vi "JKISM++ Switch VI Description Language Tool.vi"() -> ()   [LabVIEW 2014]
panel:
  in  "Double Click To Run...":i32(listbox)=-1
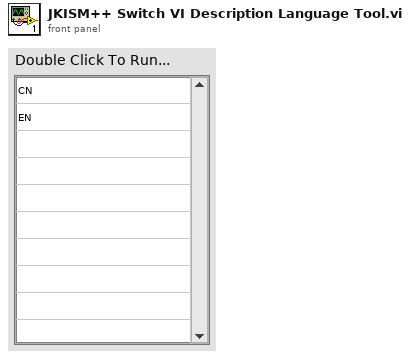
[diagram p1: front panel]
types:
  T1 = enum32{"Invalid", "Standard", "Closed", "Hidden", "Minimized", "Maximized"}
  T2 = enum32{"invalid app kind", "Development System", "Run Time System", "Student Edition", "Embedded LabVIEW", "Evaluation", "Custom"}
  T3 = cluster{"Core":cluster{"Current VI Reference":refnum<vi>, "Close Panel on Exit?":bool}, "Your Boolean data":bool, "Language":string[], "Help Root":path}
  T4 = cluster{"Current VI Reference":refnum<vi>, "Close Panel on Exit?":bool}
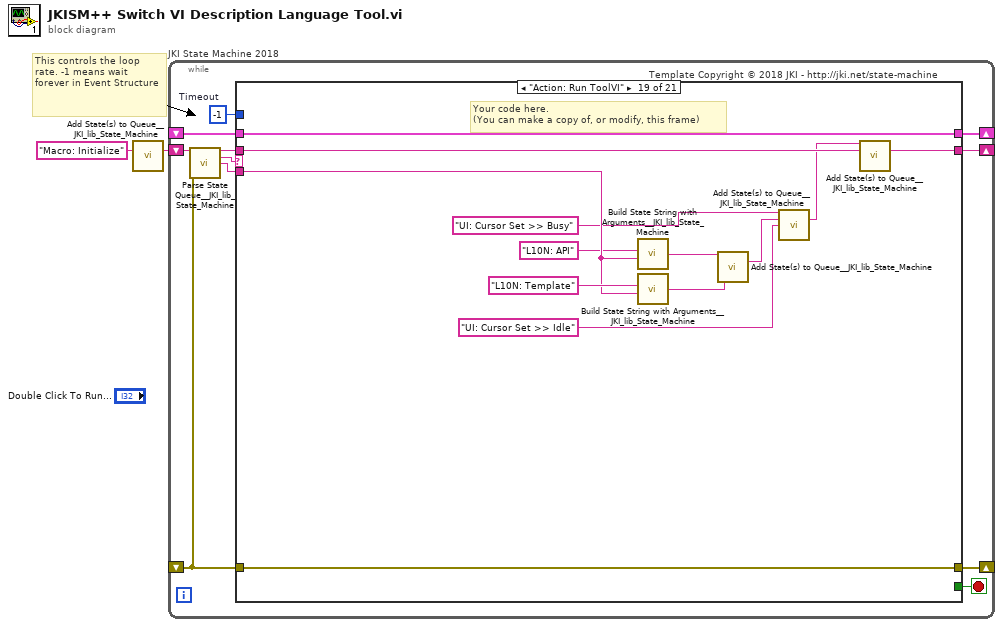
[diagram p0: block diagram]
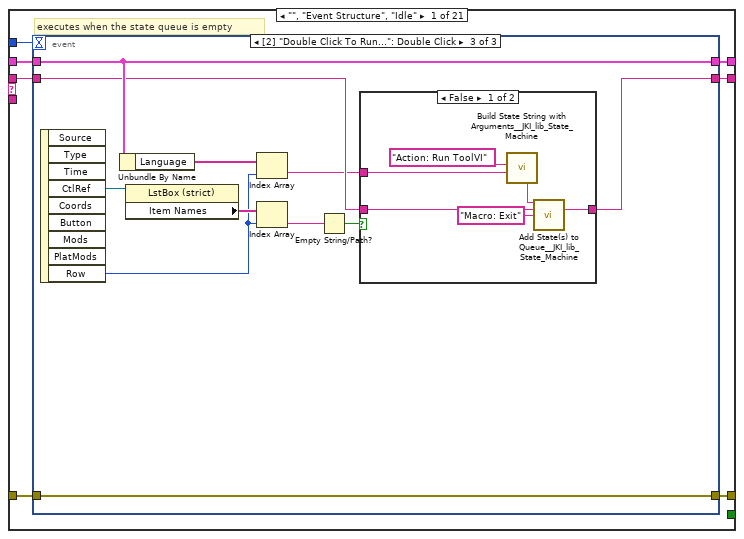
[diagram p2: hidden frame]
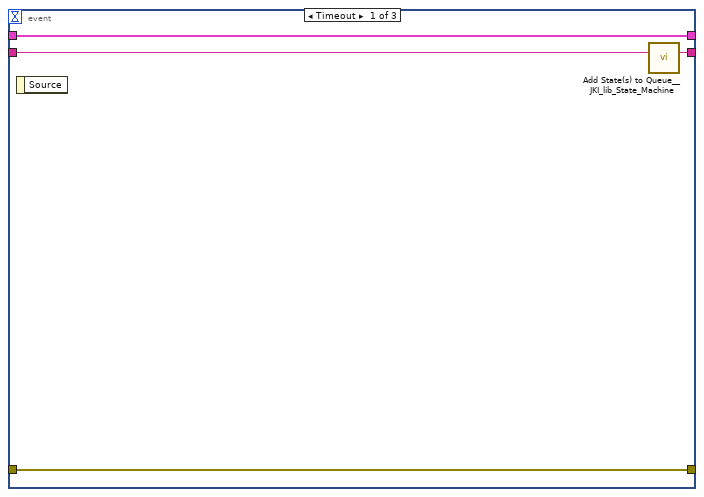
[diagram p3: hidden frame]
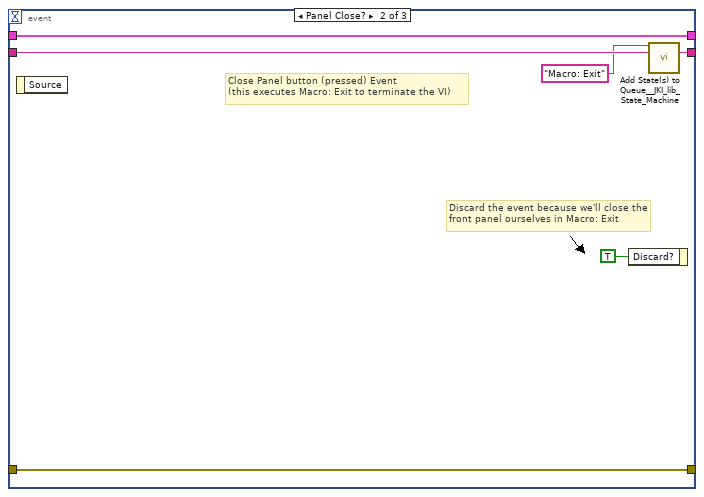
[diagram p4: hidden frame]
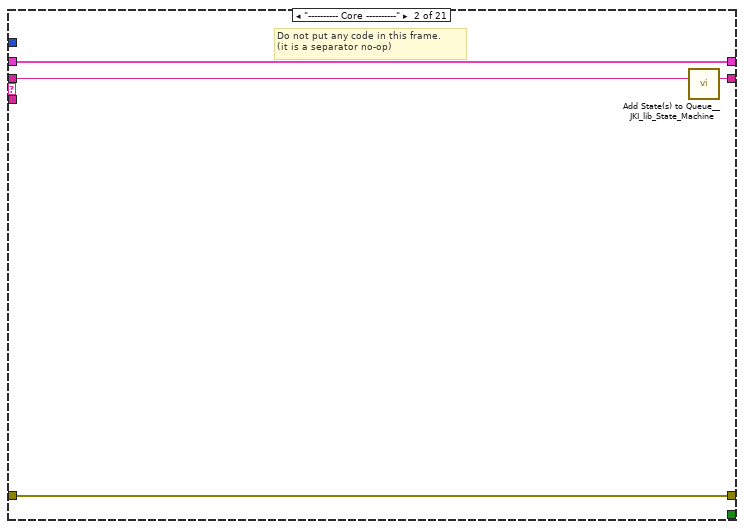
[diagram p6: hidden frame]
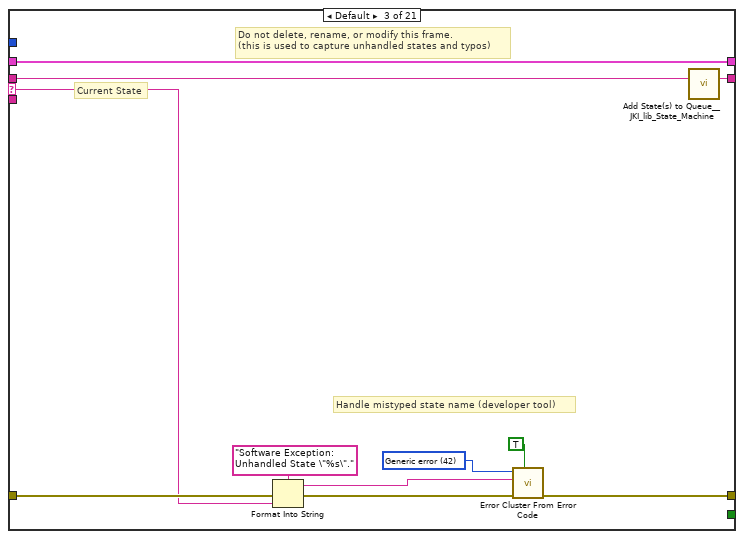
[diagram p7: hidden frame]
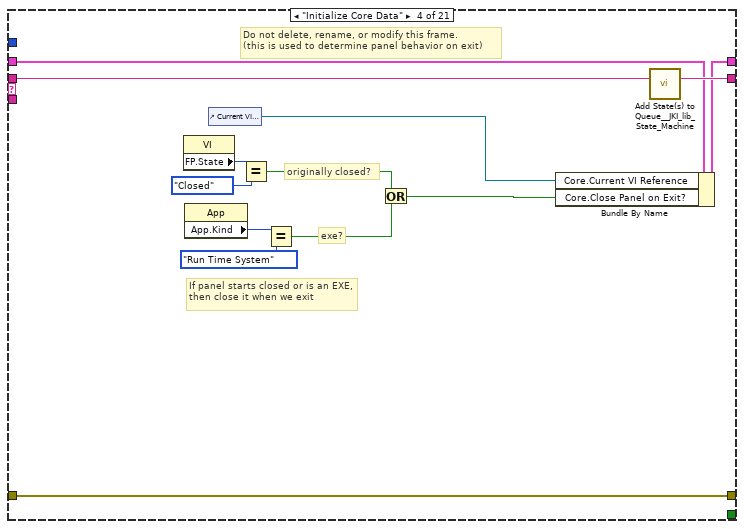
[diagram p8: hidden frame]
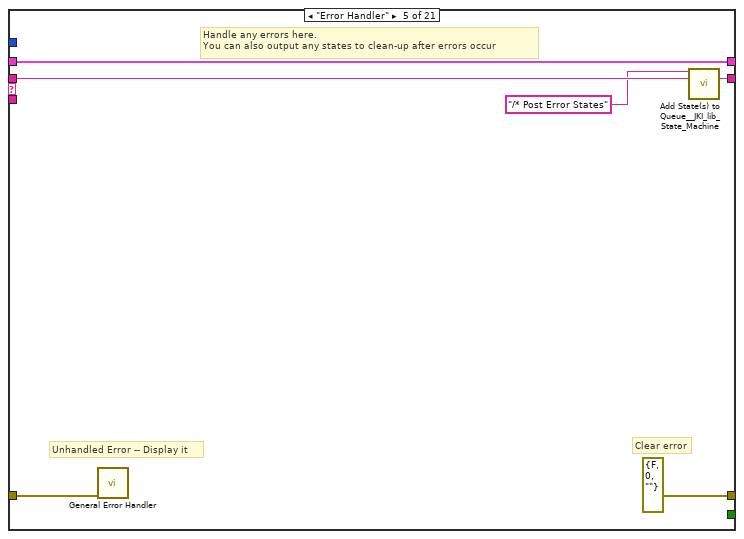
[diagram p9: hidden frame]
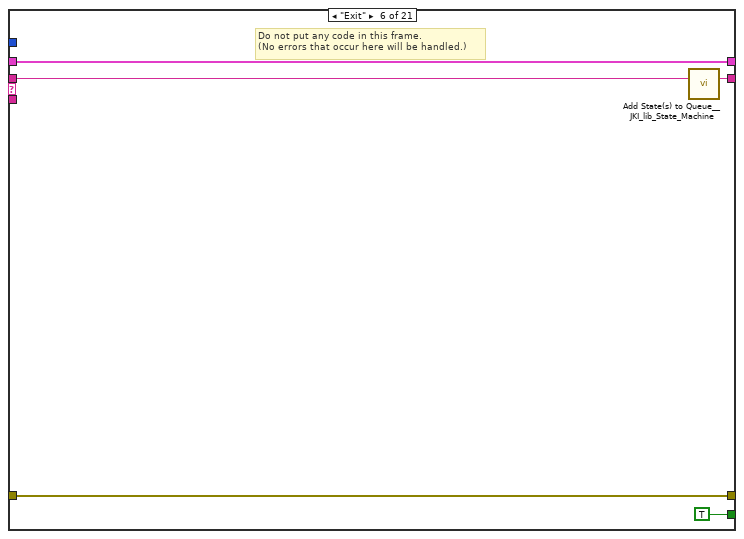
[diagram p10: hidden frame]
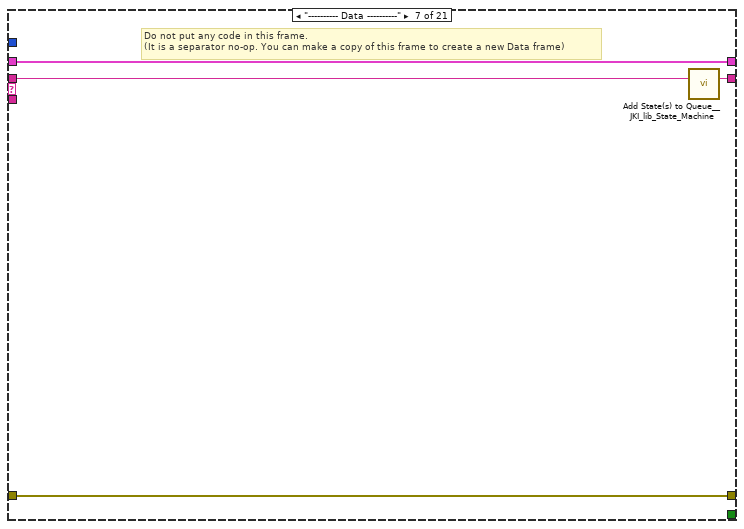
[diagram p11: hidden frame]
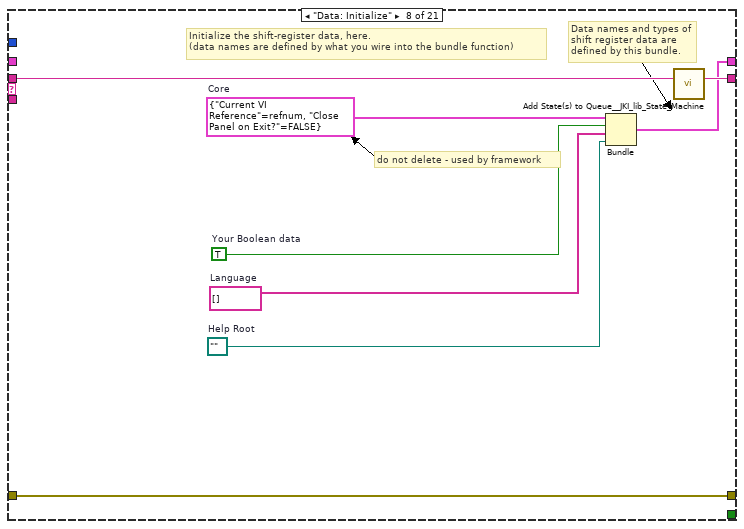
[diagram p12: hidden frame]
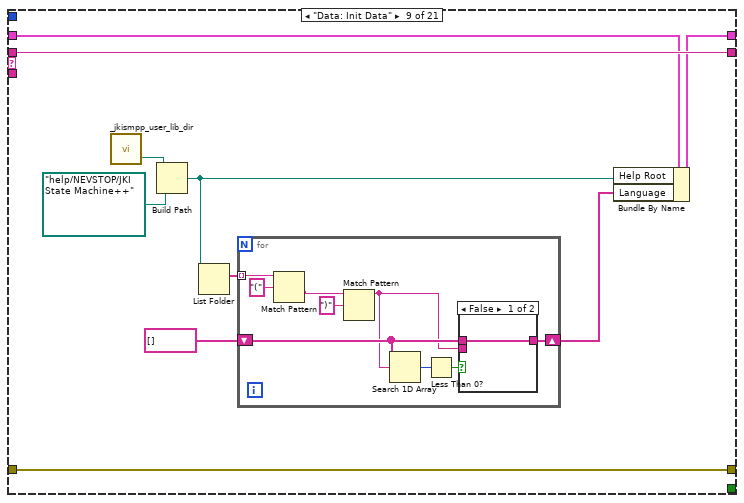
[diagram p13: hidden frame]
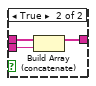
[diagram p14: hidden frame]
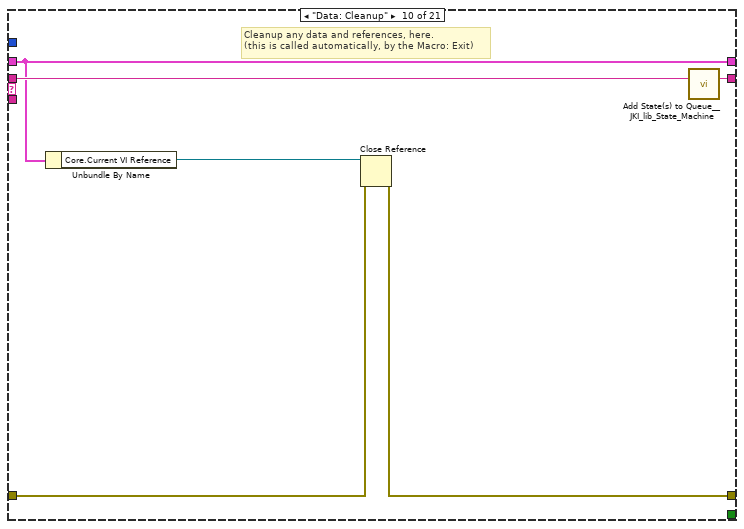
[diagram p15: hidden frame]
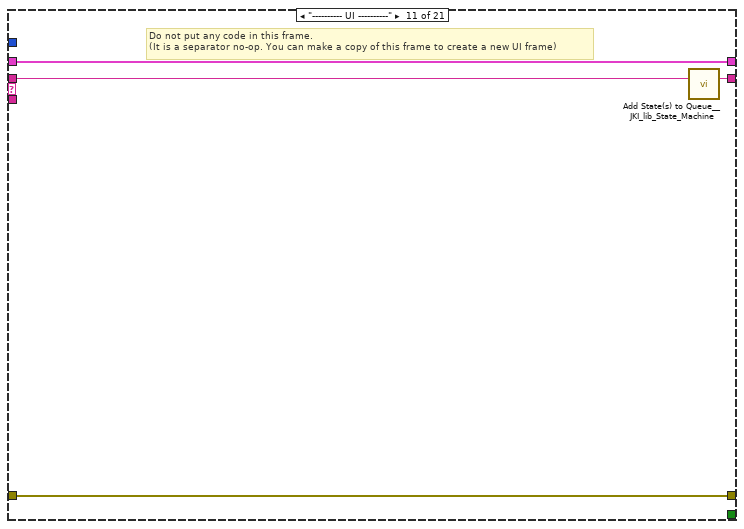
[diagram p16: hidden frame]
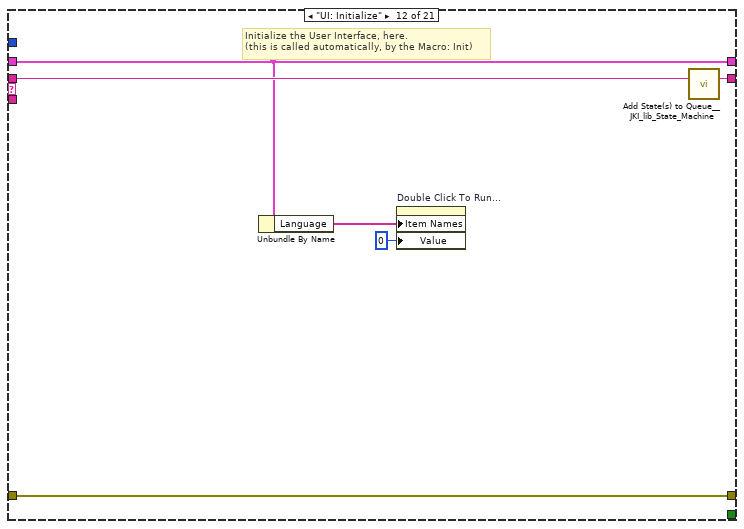
[diagram p17: hidden frame]
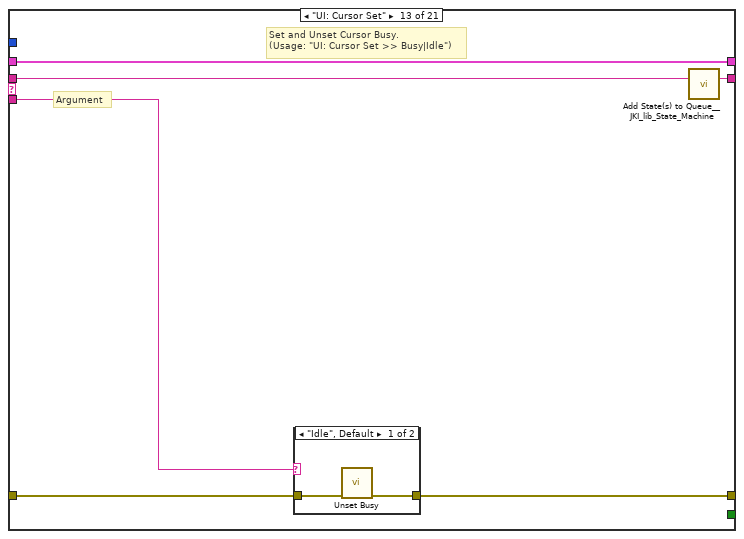
[diagram p18: hidden frame]
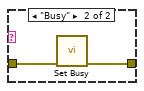
[diagram p19: hidden frame]
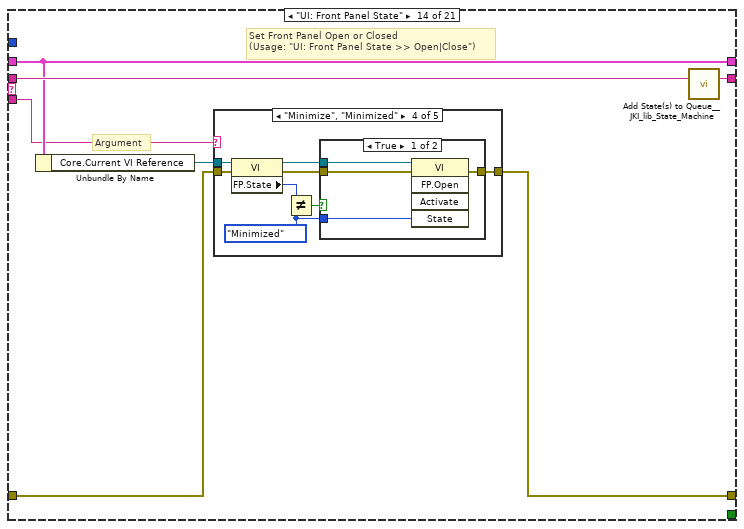
[diagram p20: hidden frame]
diagram:
  # "This controls the loop rate. -1 means wait forever in Event Structure"
  n1 = call <vilib>:"Add State(s) to Queue__JKI_lib_State_Machine.vi"("State(s) in (\"\")"="Macro: Initialize") -> ("States Out"=w2:string)  [unwired: 14 in]
  n2 = while "JKI State Machine 2018" {
    shift-right: [w6] -> _
    shift-left: _ -> [w5]
    shift-right: [w9] -> _
    shift-left: _ -> [w3]
    shift-right: [w8] -> _
    shift-left: w2 -> [w10]
    stop <- w7 stop-if-true
    w4 = -1  # Timeout
    # "Template Copyright © 2018 JKI - http://jki.net/state-machine"
    n3 = call <vilib>:"Parse State Queue__JKI_lib_State_Machine.vi"("State Queue"=w10, "Error In (no error)"=w3) -> ("Remaining States"=w12:string, "Current State"=w13:string, "Arguments"=w11:string)  [unwired: 11 in]
    n4 = case shown="\"Action: Run ToolVI\"" w13 {
      selector: w13 -> [_ _ w53 _ _ _ _ _ _ _ _ _ _ _ _ _ _ _ _ _ _]
      tunnel: w12 -> [w20 w52 w57 w76 w82 w87 w91 w99 w108 w128 w132 w138 w144 w155 w224 w229 w239 w243 w256 w266 w277]
      tunnel: w11 -> [_ _ _ _ _ _ _ _ _ _ _ _ w139 w149 _ _ _ _ w249 w257 w268]
      tunnel: w5 -> [w18 w49 w55 w69 w79 w85 w88 _ w107 w123 w129 w135 w142 w151 w221 w226 w236 w240 w254 w260 w276]
      tunnel: [w17 w50 w59 w73 errorcluster {"status"=FALSE, "code"=0, "source"=""} ("error out") w84 w89 w96 w109 w124 w130 w136 w140 w152 w222 w227 w237 w241 w253 w267 w278] -> w9
      tunnel: w3 -> [w16 w50 w58 w73 w78 w84 w89 w96 w109 w125 w130 w136 w141 w153 w222 w227 w237 w241 w253 w267 w278]
      tunnel: [w19 w51 w56 w75 w81 w86 w90 w98 w108 w127 w131 w137 w143 w154 w223 w228 w238 w242 w255 w266 w277] -> w8
      tunnel: [_ _ _ _ _ TRUE _ _ _ _ _ _ _ _ _ _ _ _ _ _ _] -> w7
      tunnel: [w15 w49 w55 w74 w79 w85 w88 w97 w106 w123 w129 w135 w142 w151 w221 w226 w236 w240 w254 w260 w276] -> w6
      tunnel: w4 -> [w14 _ _ _ _ _ _ _ _ _ _ _ _ _ _ _ _ _ _ _ _]
      frame "", "Event Structure", "Idle" {
        # "executes when the state queue is empty"
        n5 = event shown="[2] \"Double Click To Run...\": Double Click" {
          selector: _ -> [_ _ _]
          dyn-events: _ -> [_ _ _]
          timeout: w14 -> [_ _ _]
          tunnel: w20 -> [w24 w30 w35]
          tunnel: [w23 w29 w34] -> w19
          tunnel: w18 -> [w21 w27 w38]
          tunnel: [w22 w28 w41] -> w17
          tunnel: w16 -> [w22 w28 w41]
          tunnel: [w21 w27 w38] -> w15
          event Timeout {
            n6 = event-data() -> ()  [unwired: 1 in, 1 out]
            n7 = call <vilib>:"Add State(s) to Queue__JKI_lib_State_Machine.vi"("State(s) in (\"\")"=w24) -> ("States Out"=w23:string)  [unwired: 14 in]
          }
          event Panel Close? {
            # "Discard the event because we'll close the front panel ourselves in Macro: Exit"
            # "Close Panel button (pressed) Event\n(this executes Macro: Exit to terminate the VI)"
            n8 = event-data() -> ()  [unwired: 1 in, 1 out]
            n9 = event-data("Discard?"=TRUE) -> ()  [unwired: 1 in, 1 out]
            n10 = call <vilib>:"Add State(s) to Queue__JKI_lib_State_Machine.vi"("State(s) in Front (\"\")"="Macro: Exit", "State(s) in (\"\")"=w30) -> ("States Out"=w29:string)  [unwired: 13 in]
          }
          event "Double Click To Run...": Double Click {
            n11 = event-data() -> ("CtlRef"=w40:refnum<vi>, "Row"=w36:i32)  [unwired: 1 in, 7 out]
            n12 = Unbundle By Name(w38) -> ("Language"=w37:string[])
            n13 = property class="LstBox (strict)"(reference=w40) -> ("Item Names"=w39:string[])  [unwired: 1 in, 2 out]
            n14 = Index Array(array=w37, index=w36) -> (element=w31:string)
            n15 = Index Array(array=w39, index=w36) -> (element=w33:string)
            n16 = Empty String/Path?(string/path=w33) -> (empty?=w32:bool)
            n17 = case shown="False" w32 {
              tunnel: w35 -> [w47 w48]
              tunnel: [w46 w48] -> w34
              tunnel: w31 -> [w42 _]
              frame False {
                n18 = call <vilib>:"Build State String with Arguments__JKI_lib_State_Machine.vi"("Arguments (\"\")"=w42, "State"="Action: Run ToolVI") -> ("State with Arguments"=w44:string)  [unwired: 4 in]
                n19 = call <vilib>:"Add State(s) to Queue__JKI_lib_State_Machine.vi"("State(s) in Front (\"\")"=w44, "State(s) in (\"\")"=w47, "State(s) at Back (\"\")"="Macro: Exit" ("State(s) at Back (\"\")")) -> ("States Out"=w46:string)  [unwired: 12 in]
              }
              frame True {
              }
            }
          }
        }
      }
      frame "---------- Core ----------" {
        # "Do not put any code in this frame.\n(it is a separator no-op)"
        n20 = call <vilib>:"Add State(s) to Queue__JKI_lib_State_Machine.vi"("State(s) in (\"\")"=w52) -> ("States Out"=w51:string)  [unwired: 14 in]
      }
      frame Default {
        w62 = 42 items=["No error", "Argument error", "Memory is full", "Out of zone", "End of file", "File already open", "Generic file I/O error", "File not found", "File permission error", "Disk is full", "Duplicate path", "Too many files open", "System feature not enabled", "Resource file not found", "Cannot add resource", "Resource not found", "Image not found", "Image memory error", "Pen does not exist", "Config type invalid", "Config token not found", "Config parse error", "Config memory error", "Bad external code format", "Bad external code offset", "External code not present", "Null window", "Destroy window error", "Null menu", "Print aborted", "Bad print record", "Print driver error", "Windows error during printing", "Memory error during printing", "Print dialog error", "Generic print error", "Invalid device refnum", "Device not found", "Device parameter error", "Device unit error", "Cannot open device", "Device call aborted", "Generic error", "Cancelled by user", "Object ID too low", "Object ID too high", "Object not in heap", "Unknown heap", "Unknown object (invalid DefProc)", "Unknown object (DefProc not in table)", "Message out of range", "Invalid (null) method", "Unknown message", "Manager call not supported", "Bad address", "Network operation in progress", "Network operation timed out", "Connection is busy", "Network attribute not supported", "Network error", "Address in use", "System out of memory", "Connection aborted", "Connection refused", "Not connected", "Already connected", "Connection closed", "Initialization error (interapplication manager)", "Bad occurrence", "Wait on unbound occurrence handler", "Occurrence queue overflow", "Datalog type conflict", "Unused", "Unrecognized type (interapplication manager)", "Memory corrupt", "Failed to make temporary DLL", "Old CIN version", "Drag socket not found", "Failed to load drop-object", "Failed to register OLE object", "Failed to release OLE object", "Format specifier type mismatch", "Unknown format specifier", "Too few format specifiers", "Too many format specifiers", "Scan failed", "Newer CIN version", "Error converting to variant", "Runtime menu error", "Password tampered", "Variant attribute not found", "Incompatible variant data type", "Event data is not available", "Event Store is not present", "Occurrence is not found", "Event Queue is not created", "Event info is not available", "Refnum passed is NULL", "Error retrieving Class GUID", "Error retrieving CoClass GUID", "Error retrieving TypeLib GUID.", "Bad built application magic bytes.", "Specific driver is different from the specific driver associated with the Logical Name.", "There is no session opened to the class driver.", "Max Error", "MAX - Error with config objects", "MAX - Error loading configuration", "MAX - Group not supported"]
        # "Current State"
        # "Do not delete, rename, or modify this frame.\n(this is used to capture unhandled states and typos)"
        # "Handle mistyped state name (developer tool)"
        n21 = Format Into String(format string="Software Exception: Unhandled State \"%s\"." ("message"), error in=w58, w53) -> (resulting string=w61:string, error out=w60:errorcluster)  [unwired: 1 in]
        n22 = call <vilib>:"Error Cluster From Error Code.vi"("show call chain? (False)"=TRUE, "error in (no error)"=w60, "error message (\"\")"=w61, "error code (0)"=w62) -> ("error out"=w59:errorcluster)  [unwired: 5 in]
        n23 = call <vilib>:"Add State(s) to Queue__JKI_lib_State_Machine.vi"("State(s) in (\"\")"=w57) -> ("States Out"=w56:string)  [unwired: 14 in]
      }
      frame "Initialize Core Data" {
        # "Do not delete, rename, or modify this frame.\n(this is used to determine panel behavior on exit)"
        # "originally closed?"
        # "exe?"
        # "If panel starts closed or is an EXE, then close it when we exit"
        n24 = property class="VI"() -> ("FP.State"=w66:T1)  [unwired: 2 in, 2 out]
        n25 = property class="App"() -> ("App.Kind"=w72:T2)  [unwired: 2 in, 2 out]
        n26 = control-ref of="Current VI Reference"() -> (w67:refnum<vi>)
        n27 = Equal?(x=w66, y=T1."Closed" ("Front Panel Window:State")) -> (x = y?=w64:bool)
        n28 = Equal?(x=w72, y=T2."Run Time System" ("Application:Kind")) -> (x = y?=w70:bool)
        n29 = Or(x=w64, y=w70) -> (x .or. y?=w68:bool)
        n30 = Bundle By Name(cluster=w69, "Core.Current VI Reference"=w67, "Core.Close Panel on Exit?"=w68) -> (w74:T3)
        n31 = call <vilib>:"Add State(s) to Queue__JKI_lib_State_Machine.vi"("State(s) in (\"\")"=w76) -> ("States Out"=w75:string)  [unwired: 14 in]
      }
      frame "Error Handler" {
        # "Unhandled Error -- Display it"
        # "Handle any errors here.\nYou can also output any states to clean-up after errors occur"
        # "Clear error"
        n32 = call <vilib>:"General Error Handler.vi"("error in (no error)"=w78) -> ()  [unwired: 10 in, 5 out]
        n33 = call <vilib>:"Add State(s) to Queue__JKI_lib_State_Machine.vi"("State(s) in Front (\"\")"="/* Post Error States", "State(s) in (\"\")"=w82) -> ("States Out"=w81:string)  [unwired: 13 in]
      }
      frame "Exit" {
        # "Do not put any code in this frame.\n(No errors that occur here will be handled.)"
        n34 = call <vilib>:"Add State(s) to Queue__JKI_lib_State_Machine.vi"("State(s) in (\"\")"=w87) -> ("States Out"=w86:string)  [unwired: 14 in]
      }
      frame "---------- Data ----------" {
        # "Do not put any code in this frame.\n(It is a separator no-op. You can make a copy of this frame to create a new Data frame)"
        n35 = call <vilib>:"Add State(s) to Queue__JKI_lib_State_Machine.vi"("State(s) in (\"\")"=w91) -> ("States Out"=w90:string)  [unwired: 14 in]
      }
      frame "Data: Initialize" {
        w92 = string[] []  # Language
        w93 = path ""  # Help Root
        w94 = T4 {"Current VI Reference"=refnum, "Close Panel on Exit?"=FALSE}  # Core
        w95 = TRUE  # Your Boolean data
        # "do not delete - used by framework"
        # "Data names and types of shift register data are defined by this bundle."
        # "Initialize the shift-register data, here.\n(data names are defined by what you wire into the bundle function)"
        n36 = Bundle("Core"=w94, "Your Boolean data"=w95, "Language"=w92, "Help Root"=w93) -> (w97:T3)  [unwired: 1 in]
        n37 = call <vilib>:"Add State(s) to Queue__JKI_lib_State_Machine.vi"("State(s) in (\"\")"=w99) -> ("States Out"=w98:string)  [unwired: 14 in]
      }
      frame "Data: Init Data" {
        n38 = call "_jkismpp_user_lib_dir.vi"() -> ("<LabVIEW>"=w104:path)  [unwired: 2 in, 1 out]
        n39 = Build Path(base path=w104, name or relative path=path "help/NEVSTOP/JKI State Machine++" ("Path")) -> (appended path=w103:path)
        n40 = List Folder(path=w103) -> (filenames=w102:string[])  [unwired: 3 in, 3 out]
        n41 = for {
          tunnel: w102 -> [w118] mode=indexing
          shift-right: [w113] -> w100
          shift-left: string[] [] -> [w114]
          n42 = Match Pattern(string=w118, regular expression="(") -> (after substring=w115:string)  [unwired: 1 in, 3 out]
          n43 = Match Pattern(string=w115, regular expression=")") -> (before substring=w112:string)  [unwired: 1 in, 3 out]
          n44 = Search 1D Array(1D array=w114, element=w112) -> (index of element=w111:i32)  [unwired: 1 in]
          n45 = Less Than 0?(x=w111) -> (x < 0?=w110:bool)
          n46 = case shown="False" w110 {
            tunnel: w114 -> [w119 w122]
            tunnel: [w119 w121] -> w113
            tunnel: w112 -> [_ w120]
            frame False {
            }
            frame True {
              n47 = Build Array (concatenate)(w122, w120) -> (w121:string[])
            }
          }
        }
        n48 = Bundle By Name(cluster=w107, "Help Root"=w103, "Language"=w100) -> (w106:T3)
      }
      frame "Data: Cleanup" {
        # "Cleanup any data and references, here.\n(this is called automatically, by the Macro: Exit)"
        n49 = Unbundle By Name(w123) -> ("Core.Current VI Reference"=w126:refnum<vi>)
        n50 = Close Reference(reference=w126, error in (no error)=w125) -> (error out=w124:errorcluster)
        n51 = call <vilib>:"Add State(s) to Queue__JKI_lib_State_Machine.vi"("State(s) in (\"\")"=w128) -> ("States Out"=w127:string)  [unwired: 14 in]
      }
      frame "---------- UI ----------" {
        # "Do not put any code in this frame.\n(It is a separator no-op. You can make a copy of this frame to create a new UI frame)"
        n52 = call <vilib>:"Add State(s) to Queue__JKI_lib_State_Machine.vi"("State(s) in (\"\")"=w132) -> ("States Out"=w131:string)  [unwired: 14 in]
      }
      frame "UI: Initialize" {
        # "Initialize the User Interface, here.\n(this is called automatically, by the Macro: Init)"
        n53 = Unbundle By Name(w135) -> ("Language"=w134:string[])
        n54 = property on="Double Click To Run..." class="LstBox (strict)"("Item Names"=w134, "Value"=0 ("Double Click To Run...")) -> ()  [unwired: 2 in, 2 out]
        n55 = call <vilib>:"Add State(s) to Queue__JKI_lib_State_Machine.vi"("State(s) in (\"\")"=w138) -> ("States Out"=w137:string)  [unwired: 14 in]
      }
      frame "UI: Cursor Set" {
        # "Argument"
        # "Set and Unset Cursor Busy.\n(Usage: \"UI: Cursor Set >> Busy|Idle\")"
        n56 = case shown="\"Idle\", Default" w139 {
          tunnel: w141 -> [w146 w148]
          tunnel: [w145 w147] -> w140
          frame "Idle", Default {
            n57 = call <vilib>:"Unset Busy.vi"("error in (no error)"=w146) -> ("error out"=w145:errorcluster)  [unwired: 10 in]
          }
          frame "Busy" {
            n58 = call <vilib>:"Set Busy.vi"("error in (no error)"=w148) -> ("error out"=w147:errorcluster)  [unwired: 9 in, 1 out]
          }
        }
        n59 = call <vilib>:"Add State(s) to Queue__JKI_lib_State_Machine.vi"("State(s) in (\"\")"=w144) -> ("States Out"=w143:string)  [unwired: 14 in]
      }
      frame "UI: Front Panel State" {
        # "Argument"
        # "Set Front Panel Open or Closed\n(Usage: \"UI: Front Panel State >> Open|Close\")"
        n60 = Unbundle By Name(w151) -> ("Core.Current VI Reference"=w150:refnum<vi>)
        n61 = case shown="\"Minimize\", \"Minimized\"" w149 {
          tunnel: w153 -> [w161 w176 w187 w200 w213]
          tunnel: [w163 w177 w189 w202 w215] -> w152
          tunnel: w150 -> [w162 w174 w188 w201 w214]
          frame "Open", "Standard", Default {
            w156 = T1."Standard" ("State")
            n62 = property class="VI"(reference=w162, error in=w161) -> (reference out=w159:refnum<vi>, error out=w160:errorcluster, "FP.State"=w158:T1)
            n63 = Not Equal?(x=w158, y=w156) -> (x != y?=w157:bool)
            n64 = case shown="True" w157 {
              tunnel: [w167 w169] -> w163
              tunnel: w160 -> [w166 w169]
              tunnel: w159 -> [w165 _]
              tunnel: w156 -> [w164 _]
              frame True {
                n65 = invoke class="VI" method="FP.Open"(reference=w165, error in=w166, "Activate"=TRUE, "State"=w164) -> (error out=w167:errorcluster)  [unwired: 1 in, 4 out]
              }
              frame False {
              }
            }
          }
          frame "Close", "Closed" {
            n66 = property class="VI"(reference=w174, error in=w176) -> (reference out=w173:refnum<vi>, error out=w175:errorcluster, "FP.State"=w171:T1)
            n67 = Not Equal?(x=w171, y=T1."Closed" ("Front Panel Window:State")) -> (x != y?=w170:bool)
            n68 = case shown="True" w170 {
              tunnel: [w178 w181] -> w177
              tunnel: w175 -> [w178 w180]
              tunnel: w173 -> [_ w179]
              frame False {
              }
              frame True {
                n69 = invoke class="VI" method="FP.Close"(reference=w179, error in=w180) -> (error out=w181:errorcluster)  [unwired: 1 in, 2 out]
              }
            }
          }
          frame "Hidden", "Hide" {
            w182 = T1."Hidden" ("State")
            n70 = property class="VI"(reference=w188, error in=w187) -> (reference out=w185:refnum<vi>, error out=w186:errorcluster, "FP.State"=w184:T1)
            n71 = Not Equal?(x=w184, y=w182) -> (x != y?=w183:bool)
            n72 = case shown="True" w183 {
              tunnel: [w193 w194] -> w189
              tunnel: w186 -> [w192 w194]
              tunnel: w185 -> [w191 _]
              tunnel: w182 -> [w190 _]
              frame True {
                n73 = invoke class="VI" method="FP.Open"(reference=w191, error in=w192, "State"=w190) -> (error out=w193:errorcluster)  [unwired: 2 in, 4 out]
              }
              frame False {
              }
            }
          }
          frame "Minimize", "Minimized" {
            w195 = T1."Minimized" ("State")
            n74 = property class="VI"(reference=w201, error in=w200) -> (reference out=w198:refnum<vi>, error out=w199:errorcluster, "FP.State"=w197:T1)
            n75 = Not Equal?(x=w197, y=w195) -> (x != y?=w196:bool)
            n76 = case shown="True" w196 {
              tunnel: [w206 w207] -> w202
              tunnel: w199 -> [w205 w207]
              tunnel: w198 -> [w204 _]
              tunnel: w195 -> [w203 _]
              frame True {
                n77 = invoke class="VI" method="FP.Open"(reference=w204, error in=w205, "State"=w203) -> (error out=w206:errorcluster)  [unwired: 2 in, 4 out]
              }
              frame False {
              }
            }
          }
          frame "Maximize", "Maximized" {
            w208 = T1."Maximized" ("State")
            n78 = property class="VI"(reference=w214, error in=w213) -> (reference out=w211:refnum<vi>, error out=w212:errorcluster, "FP.State"=w210:T1)
            n79 = Not Equal?(x=w210, y=w208) -> (x != y?=w209:bool)
            n80 = case shown="True" w209 {
              tunnel: [w219 w220] -> w215
              tunnel: w212 -> [w218 w220]
              tunnel: w211 -> [w217 _]
              tunnel: w208 -> [w216 _]
              frame True {
                n81 = invoke class="VI" method="FP.Open"(reference=w217, error in=w218, "State"=w216) -> (error out=w219:errorcluster)  [unwired: 2 in, 4 out]
              }
              frame False {
              }
            }
          }
        }
        n82 = call <vilib>:"Add State(s) to Queue__JKI_lib_State_Machine.vi"("State(s) in (\"\")"=w155) -> ("States Out"=w154:string)  [unwired: 14 in]
      }
      frame "---------- Macro ----------" {
        # "Do not put any code in this frame.\n(It is a separator no-op. You can make a copy of this frame to create a new Macro frame)"
        n83 = call <vilib>:"Add State(s) to Queue__JKI_lib_State_Machine.vi"("State(s) in (\"\")"=w224) -> ("States Out"=w223:string)  [unwired: 14 in]
      }
      frame "Macro: Initialize" {
        w225 = "Data: Initialize\nInitialize Core Data\nData: Init Data\nUI: Initialize\nUI: Front Panel State >> Open"  # Data: Initialize Initialize Core Data Data: Init Data UI: Initialize UI: Front Panel State >> Open
        # "Initialization Macro\n(This is called once, when the VI starts)"
        n84 = call <vilib>:"Add State(s) to Queue__JKI_lib_State_Machine.vi"("State(s) in Front (\"\")"=w225, "State(s) in (\"\")"=w229) -> ("States Out"=w228:string)  [unwired: 13 in]
      }
      frame "Macro: Exit" {
        # "Exit Macro\n(This is called once, when the VI exits)"
        n85 = Unbundle By Name(w236) -> ("Core.Close Panel on Exit?"=w235:bool)
        n86 = Select(t="UI: Front Panel State >> Close", s=w235, f="") -> (s? t:f=w232:string)
        n87 = call <vilib>:"Add State(s) to Queue__JKI_lib_State_Machine.vi"("State(s) in (\"\")"=w232, "State(s) at Back (\"\")"="Data: Cleanup\nExit") -> ("States Out"=w230:string)  [unwired: 13 in]
        n88 = call <vilib>:"Add State(s) to Queue__JKI_lib_State_Machine.vi"("State(s) in Front (\"\")"=w230, "State(s) in (\"\")"=w239) -> ("States Out"=w238:string)  [unwired: 13 in]
      }
      frame "---------- Action ----------" {
        # "Template Separator\n(You can make a copy of, or modify, this frame)"
        n89 = call <vilib>:"Add State(s) to Queue__JKI_lib_State_Machine.vi"("State(s) in (\"\")"=w243) -> ("States Out"=w242:string)  [unwired: 14 in]
      }
      frame "Action: Run ToolVI" {
        # "Your code here.\n(You can make a copy of, or modify, this frame)"
        n90 = call <vilib>:"Build State String with Arguments__JKI_lib_State_Machine.vi"("Arguments (\"\")"=w249, "State"="L10N: API" ("State(s) in Front (\"\")")) -> ("State with Arguments"=w252:string)  [unwired: 4 in]
        n91 = call <vilib>:"Build State String with Arguments__JKI_lib_State_Machine.vi"("Arguments (\"\")"=w249, "State"="L10N: Template" ("State(s) in Front (\"\")")) -> ("State with Arguments"=w251:string)  [unwired: 4 in]
        n92 = call <vilib>:"Add State(s) to Queue__JKI_lib_State_Machine.vi"("State(s) in Front (\"\")"=w252, "State(s) at Back (\"\")"=w251) -> ("States Out"=w247:string)  [unwired: 13 in]
        n93 = call <vilib>:"Add State(s) to Queue__JKI_lib_State_Machine.vi"("State(s) in Front (\"\")"="UI: Cursor Set >> Busy" ("State(s) in Front (\"\")"), "State(s) in (\"\")"=w247, "State(s) at Back (\"\")"="UI: Cursor Set >> Idle" ("State(s) in Front (\"\")")) -> ("States Out"=w246:string)  [unwired: 12 in]
        n94 = call <vilib>:"Add State(s) to Queue__JKI_lib_State_Machine.vi"("State(s) in Front (\"\")"=w246, "State(s) in (\"\")"=w256) -> ("States Out"=w255:string)  [unwired: 13 in]
      }
      frame "L10N: API" {
        n95 = Unbundle By Name(w260) -> ("Help Root"=w261:path)  [unwired: 1 out]
        n96 = Concatenate Strings("VI Description" ("string"), "(" ("string"), w257, ")" ("string"), ".md" ("string")) -> (w262:string)
        n97 = Build Path(base path=w261, name or relative path=w262) -> (appended path=w259:path)
        n98 = call "_script_import_api_doc.vi"("md path"=w259) -> ()  [unwired: 11 in]
      }
      frame "L10N: Template" {
        n99 = Unbundle By Name(w276) -> ("Help Root"=w271:path)  [unwired: 1 out]
        n100 = Concatenate Strings("Template Description" ("string"), "(" ("string"), w268, ")" ("string"), ".md" ("string")) -> (w272:string)
        n101 = Build Path(base path=w271, name or relative path=w272) -> (appended path=w270:path)
        n102 = call "_script_import_template_doc.vi"("md path"=w270) -> ()  [unwired: 11 in]
      }
    }
  }
